vi "CANOpen_Initialize VS NMT Data Refs.vi"(6 "Name":string, 7 "Node indexes":dbl[](array[numeric]), 8 "error in (no error)":errorcluster, 9 "Hardware Output Refs":T1[](array[typedef]) format="%.0x", 10 "Hardware Input Refs":T1[][](array[typedef]) format="%.0x", 11 "Device Ref":T1 format="%.0x") -> (0 "error out":errorcluster, 2 "Data References":T2 {"Hardware Output"."Channel Pairs"."Chan Refs"."Data Reference" format="%.0x"; "Hardware Input"."Channel Pairs"."Chan Refs" format="%.0x"})   [LabVIEW 2013, in "CANOpen Addon Custom Device.lvlib"]
uses:
  CANOpen Addon Custom Device.lvlib
  CANOpen_VS Status Management Data Refs.ctl
  Async VIs/CANOpen_Main/SubVIs/CanOpen_NMT_HWOut_ChannelPairs.ctl
  <vilib>/NI Veristand/Custom Device API/Block Data Reference.ctl
  <vilib>/NI Veristand/Custom Device API/Data Reference.ctl
  Async VIs/CANOpen_Main/SubVIs/CanOpen_NMT_HWIn_ChannelPairs.ctl
  <vilib>/NI Veristand/Custom Device API/Custom Device Item Ref.ctl
  <vilib>/NI Veristand/Custom Device API/Data Access Type.ctl
  <vilib>/NI Veristand/Custom Device API/Custom Device API.lvlib
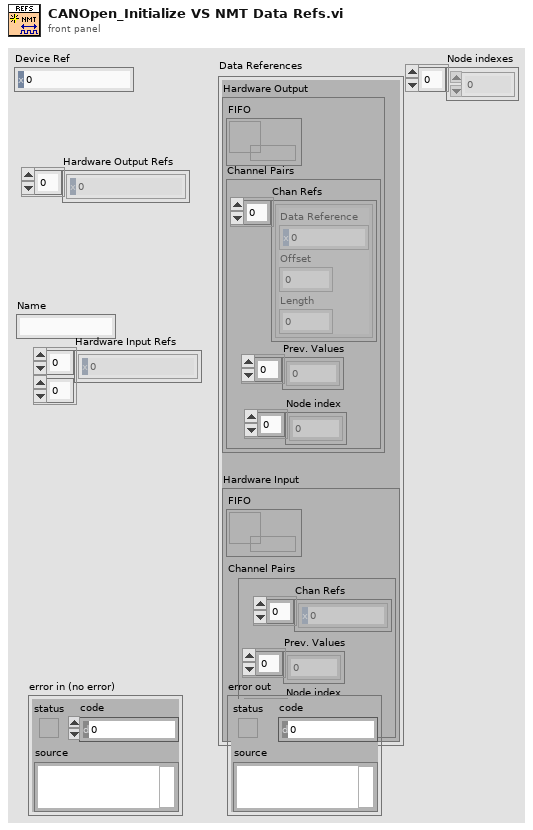
[diagram p1: front panel]
types:
  T1 = typedef "Custom Device API.lvlib/Custom Device Item Ref.ctl" = u64
  T2 = typedef "CANOpen Addon Custom Device.lvlib/CANOpen_VS Status Management Data Refs.ctl" = cluster{"Hardware Output":cluster{"FIFO":refnum<k33>, "Channel Pairs":T3}, "Hardware Input":cluster{"FIFO":refnum<k33>, "Channel Pairs":T6}}
  T3 = typedef "CANOpen Addon Custom Device.lvlib/CanOpen_NMT_HWOut_ChannelPairs.ctl" = cluster{"Chan Refs":T4[], "Prev. Values":dbl[], "Node index":dbl[]}
  T4 = typedef "Custom Device API.lvlib/Block Data Reference.ctl" = cluster{"Data Reference":T5, "Offset":i32, "Length":i32}
  T5 = typedef "Custom Device API.lvlib/Data Reference.ctl" = i32
  T6 = typedef "CANOpen Addon Custom Device.lvlib/CanOpen_NMT_HWIn_ChannelPairs.ctl" = cluster{"Chan Refs":T5[], "Prev. Values":dbl[], "Node index":dbl[]}
  T7 = cluster{"read mode":enum16{"polling", "blocking"}, "write mode":enum16{"polling", "blocking"}}
  T8 = typedef "Custom Device API.lvlib/Data Access Type.ctl" = enum16{"Read", "Write"}
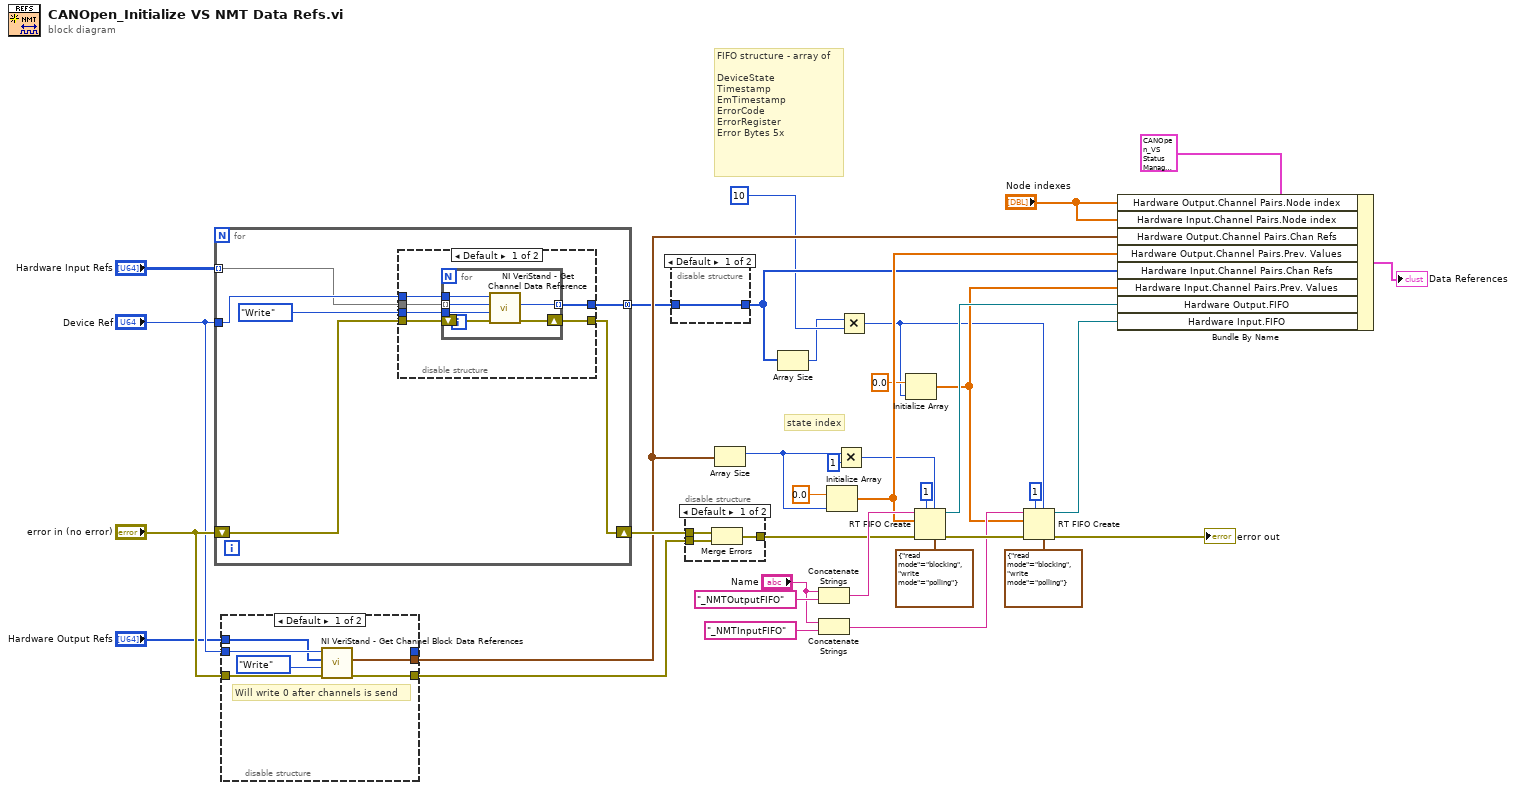
[diagram p0: block diagram]
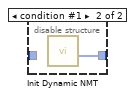
[diagram p3: hidden frame]
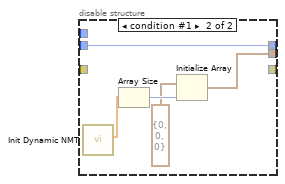
[diagram p4: hidden frame]
diagram:
  # "FIFO structure - array of\n\nDeviceState\nTimestamp\nEmTimestamp\nErrorCode\nErrorRegister\nError Bytes 5x"
  # "state index"
  n1 = for {
    shift-right: [w41] -> w19
    shift-left: "error in (no error)" -> [w37]
    tunnel: "Hardware Input Refs" -> [w40] mode=indexing
    tunnel: "Device Ref" -> [w42]
    tunnel: [w38] -> w8 mode=concatenating
    n2 = disable-structure shown="Default" {
      disable-tunnel: [w48 w55] -> w38
      disable-tunnel: Data_Access_Type."Write" ("Access") -> [w47 _]
      disable-tunnel: w42 -> [w43 _]
      disable-tunnel: w37 -> [w46 w56]
      disable-tunnel: w40 -> [w45 w55]
      disable-tunnel: [w44 w56] -> w41
      frame condition #0 (active) {
        n3 = for {
          tunnel: w45 -> [w52] mode=indexing
          tunnel: w47 -> [w51]
          shift-right: [w53] -> w44
          shift-left: w46 -> [w54]
          tunnel: [w50] -> w48 mode=indexing
          tunnel: w43 -> [w49]
          n4 = call <vilib>:"NI VeriStand - Get Channel Data Reference.vi"("error in (no error)"=w54, "Access"=w51, "Channel Ref in"=w52, "Device Ref in"=w49) -> ("error out"=w53:errorcluster, "Channel Data Reference"=w50:T5)  [unwired: 5 in, 1 out]
        }
      }
      frame condition #1 {
      }
    }
  }
  n5 = disable-structure shown="Default" {
    disable-tunnel: "Device Ref" -> [w62 w67]
    disable-tunnel: [_ w67] -> _
    disable-tunnel: [w60 _] -> w10
    disable-tunnel: "error in (no error)" -> [w59 _]
    disable-tunnel: [w61 w64] -> w13
    disable-tunnel: "Hardware Output Refs" -> [w57 _]
    frame condition #0 (active) {
      # "Will write 0 after channels is send"
      n6 = call <vilib>:"NI VeriStand - Get Channel Block Data References.vi"("error in (no error)"=w59, "Access"=Data_Access_Type."Write", "Channel Refs"=w57, "Device Ref in"=w62) -> ("error out"=w60:errorcluster, "Block Data Refs"=w61:T4[])  [unwired: 4 in, 2 out]
    }
    frame condition #1 {
      n7 = call "Init Dynamic NMT.vi"() -> ("Output"=w63:dbl[])  [unwired: 10 in, 1 out]
      n8 = Array Size(array=w63) -> (size(s)=w66:i32)
      n9 = Initialize Array(T4 {"Data Reference"=0, "Offset"=0, "Length"=0} ("Block Data Ref"), w66) -> (w64:T4[])
    }
  }
  n10 = disable-structure shown="Default" {
    disable-tunnel: [w68 w69] -> w9
    disable-tunnel: w8 -> [w68 _]
    frame condition #0 (active) {
    }
    frame condition #1 {
      n11 = call "Init Dynamic NMT.vi"() -> ("Inputs"=w69:T5[])  [unwired: 10 in, 1 out]
    }
  }
  n12 = disable-structure shown="Default" {
    disable-tunnel: w19 -> [w72 _]
    disable-tunnel: [w71 w73] -> w11
    disable-tunnel: w10 -> [w70 w73]
    frame condition #0 (active) {
      n13 = Merge Errors(w72, w70) -> (w71:errorcluster)
    }
    frame condition #1 {
    }
  }
  n14 = Array Size(array=w13) -> (size(s)=w5:i32)
  n15 = Array Size(array=w9) -> (size(s)=w2:i32)
  n16 = Concatenate Strings("Name", "_NMTOutputFIFO" ("string")) -> (w33:string)
  n17 = Concatenate Strings("Name", "_NMTInputFIFO" ("string")) -> (w23:string)
  n18 = Initialize Array(0.0 ("element"), w5) -> (w20:dbl[])
  n19 = Multiply(x=w5, y=1) -> (x*y=w4:i32)
  n20 = Multiply(x=w2, y=10) -> (x*y=w1:i32)
  n21 = Initialize Array(0.0 ("element"), w1) -> (w16:dbl[])
  n22 = RT FIFO Create(0:w33, 1:w20, 3:w11, 4:u32 1 ("size (10)"), 6:w4, 7:T7 {"read mode"=enum."blocking", "write mode"=enum."polling"} ("r/w modes (polling,polling)")) -> (8:w21:refnum<k33>, 11:w25:errorcluster)  [unwired: 2 in, 1 out]
  n23 = RT FIFO Create(0:w23, 1:w16, 3:w25, 4:u32 1 ("size (10)"), 6:w1, 7:T7 {"read mode"=enum."blocking", "write mode"=enum."polling"} ("r/w modes (polling,polling)")) -> (8:w18:refnum<k33>, 11:→"error out":errorcluster)  [unwired: 2 in, 1 out]
  n24 = Bundle By Name(cluster=T2 {"Hardware Output"={"FIFO"=refnum, "Channel Pairs"={"Chan Refs"=[], "Prev. Values"=[], "Node index"=[]}}, "Hardware Input"={"FIFO"=refnum, "Channel Pairs"={"Chan Refs"=[], "Prev. Values"=[], "Node index"=[]}}} ("Data References"), "Hardware Output.Channel Pairs.Node index"="Node indexes", "Hardware Input.Channel Pairs.Node index"="Node indexes", "Hardware Output.Channel Pairs.Chan Refs"=w13, "Hardware Output.Channel Pairs.Prev. Values"=w20, "Hardware Input.Channel Pairs.Chan Refs"=w9, "Hardware Input.Channel Pairs.Prev. Values"=w16, "Hardware Output.FIFO"=w21, "Hardware Input.FIFO"=w18) -> (→"Data References":T2)
